vi "FileVisonTest.vi"() -> ()   [LabVIEW 2011]
panel:
  out "Dist Error":dbl
  out "Angle Error":dbl
  in  "Diff in Height":dbl
  in  "Dist in Ft":dbl
  out "Elevation Angle":dbl
  out "XOR Image":T1(plugin-control)
  out "Image 2":T1(plugin-control)
  out "Image 1":T1(plugin-control)
  out "Offset Angle From Perpendicular":dbl
  out "Shortest Dist To Rect Center":dbl
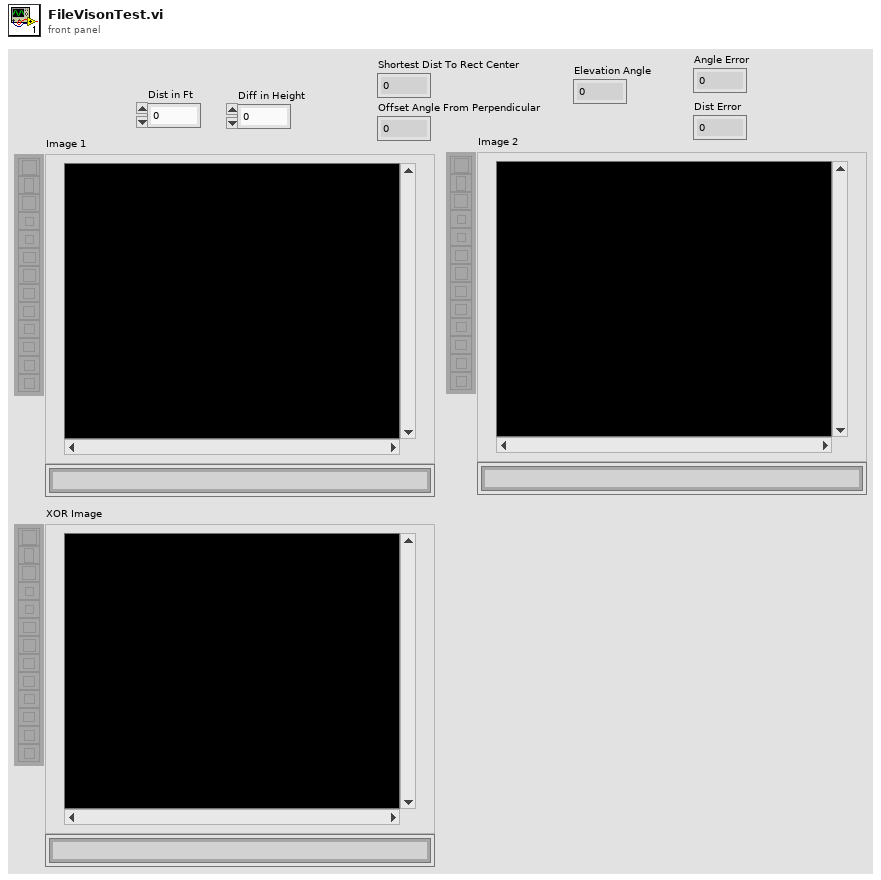
[diagram p1: front panel]
types:
  T1 = typedef "IMAQ Image.ctl" = refnum<image>
  T2 = typedef "Image Type" = u32
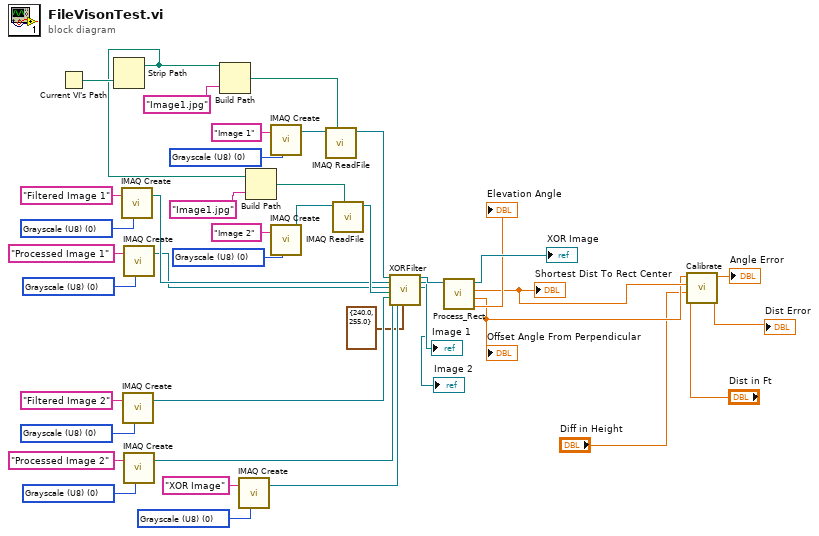
[diagram p0: block diagram]
diagram:
  w22 = T2 0 items=["Grayscale (U8)", "Grayscale (I16)", "Grayscale (SGL)", "Complex (CSG)", "RGB (U32)", "HSL (U32)", "RGB (U64)", "Grayscale (U16)"] ("Image Type")
  w23 = T2 0 items=["Grayscale (U8)", "Grayscale (I16)", "Grayscale (SGL)", "Complex (CSG)", "RGB (U32)", "HSL (U32)", "RGB (U64)", "Grayscale (U16)"] ("Image Type")
  w33 = T2 0 items=["Grayscale (U8)", "Grayscale (I16)", "Grayscale (SGL)", "Complex (CSG)", "RGB (U32)", "HSL (U32)", "RGB (U64)", "Grayscale (U16)"] ("Image Type")
  w35 = T2 0 items=["Grayscale (U8)", "Grayscale (I16)", "Grayscale (SGL)", "Complex (CSG)", "RGB (U32)", "HSL (U32)", "RGB (U64)", "Grayscale (U16)"] ("Image Type")
  w36 = T2 0 items=["Grayscale (U8)", "Grayscale (I16)", "Grayscale (SGL)", "Complex (CSG)", "RGB (U32)", "HSL (U32)", "RGB (U64)", "Grayscale (U16)"] ("Image Type")
  w39 = T2 0 items=["Grayscale (U8)", "Grayscale (I16)", "Grayscale (SGL)", "Complex (CSG)", "RGB (U32)", "HSL (U32)", "RGB (U64)", "Grayscale (U16)"] ("Image Type")
  w40 = T2 0 items=["Grayscale (U8)", "Grayscale (I16)", "Grayscale (SGL)", "Complex (CSG)", "RGB (U32)", "HSL (U32)", "RGB (U64)", "Grayscale (U16)"] ("Image Type")
  n1 = Current VI's Path() -> (path=w9:path)
  n2 = Strip Path(path=w9) -> (stripped path=w8:path)  [unwired: 1 out]
  n3 = call "IMAQ Create"("Image Name"="Filtered Image 1", "Image Type"=w36) -> ("New Image"=w19:T1)  [unwired: 3 in, 1 out]
  n4 = call "IMAQ Create"("Image Name"="Filtered Image 2", "Image Type"=w35) -> ("New Image"=w17:T1)  [unwired: 3 in, 1 out]
  n5 = call "IMAQ Create"("Image Name"="Processed Image 1", "Image Type"=w40) -> ("New Image"=w18:T1)  [unwired: 3 in, 1 out]
  n6 = call "IMAQ Create"("Image Name"="Processed Image 2", "Image Type"=w39) -> ("New Image"=w16:T1)  [unwired: 3 in, 1 out]
  n7 = Build Path(base path=w8, name or relative path="Image1.jpg") -> (appended path=w29:path)
  n8 = call "IMAQ Create"("Image Name"="XOR Image", "Image Type"=w33) -> ("New Image"=w15:T1)  [unwired: 3 in, 1 out]
  n9 = Build Path(base path=w8, name or relative path="Image1.jpg") -> (appended path=w26:path)
  n10 = call "IMAQ Create"("Image Name"="Image 1", "Image Type"=w23) -> ("New Image"=w27:T1)  [unwired: 3 in, 1 out]
  n11 = call "IMAQ Create"("Image Name"="Image 2", "Image Type"=w22) -> ("New Image"=w24:T1)  [unwired: 3 in, 1 out]
  n12 = call "IMAQ ReadFile"("File Path"=w29, "Image"=w27) -> ("Image Out"=w21:T1)  [unwired: 5 in, 4 out]
  n13 = call "IMAQ ReadFile"("File Path"=w26, "Image"=w24) -> ("Image Out"=w20:T1)  [unwired: 5 in, 4 out]
  n14 = call "XORFilter.vi"("Image Src 1"=w21, "Filtered Image Dst 1"=w19, 2:"Processed Image Dst 2"=w18, "Image Src 2"=w20, "Filtered Image Dst 2"=w17, 5:"Processed Image Dst 2"=w16, "XOR Image Dst"=w15, "Threshold Range"=cluster{"Lower value":sgl, "Upper value":sgl} {"Lower value"=240.0, "Upper value"=255.0}) -> ("XOR Image Dst Out"=w13:T1, "Image Dst 1 Out"=→"Image 1":T1, "Image Dst 2 Out"=→"Image 2":T1)  [unwired: 9 in]
  n15 = call "Process_Rect.vi"("XOR Image"=w13) -> ("Elevation Angle"=→"Elevation Angle":dbl, "Offset Angle From Perpendicular"=w5:dbl, "Shortest Dist To Rect Center"=w6:dbl, "Processed Image Out"=→"XOR Image":T1)  [unwired: 7 in]
  "Shortest Dist To Rect Center" <- w6
  "Offset Angle From Perpendicular" <- w5
  n16 = call "Calibrate.vi"("Dist in Ft"="Dist in Ft", "Diff in Height"="Diff in Height", "Calculated Dist"=w6, "Calculated Angle"=w5) -> ("Dist Error"=→"Dist Error":dbl, "Angle Error"=→"Angle Error":dbl)  [unwired: 6 in]
